vi "ThrottleMixer.vi"(9 "Input Z":dbl, 10 "Input Y":dbl, 11 "Input X":dbl) -> (0 "Rear Right Output":dbl, 1 "Rear Left Output":dbl, 2 "Front Right Output":dbl, 3 "Front Left Output":dbl)   [LabVIEW 2014]
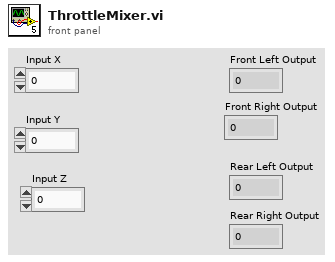
[diagram p1: front panel]
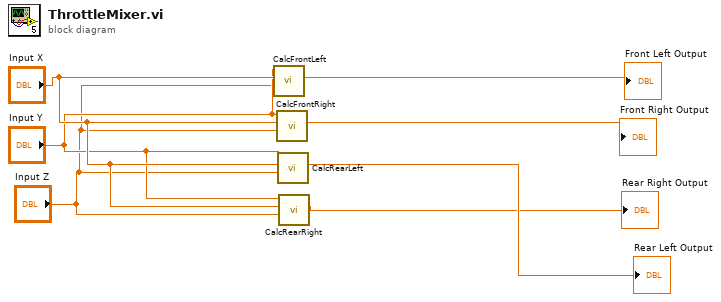
[diagram p0: block diagram]
diagram:
  n1 = call "CalcFrontLeft.vi"("Rotate Clockwise\n(Input)"="Input Z", "Strafe Left\n(Input)"="Input X", "Forward\n(Input)"="Input Y") -> ("Motor Speed\n(Output)"=→"Front Left Output":dbl)  [unwired: 8 in]
  n2 = call "CalcFrontRight.vi"("Rotate Clockwise\n(Input)"="Input Z", "Strafe Left\n(Input)"="Input X", "Forward\n(Input)"="Input Y") -> ("Motor Speed\n(Output)"=→"Front Right Output":dbl)  [unwired: 8 in]
  n3 = call "CalcRearLeft.vi"("Rotate Clockwise\n(Input)"="Input Z", "Strafe Left\n(Input)"="Input X", "Forward\n(Input)"="Input Y") -> ("Motor Speed\n(Output)"=→"Rear Left Output":dbl)  [unwired: 8 in]
  n4 = call "CalcRearRight.vi"("Rotate Clockwise\n(Input)"="Input Z", "Strafe Left\n(Input)"="Input X", "Forward\n(Input)"="Input Y") -> ("Motor Speed\n(Output)"=→"Rear Right Output":dbl)  [unwired: 8 in]
